vi "Model.vi"(7 "Throttle":dbl, 8 "Turbulance":bool, 9 "dt (s)":dbl=1.0 format="%0.2f", 10 "Motor 4":dbl=-2e-06, 11 "Motor 2":dbl=-2e-06) -> (2 "Position":cluster{"X":dbl, "Y":dbl, "Z":dbl}={"X"=0.0, "Y"=0.0, "Z"=-100.0}, 3 "Angle (degs)":dbl)   [LabVIEW 2011]
uses:
  <vilib>/ptbypt/NI_PtbyPt.lvlib
panel:
  out "M4 Torque":dbl(knob) scale=0.0..3.0
  out "M2 Torque":dbl(knob) scale=0.0..3.0
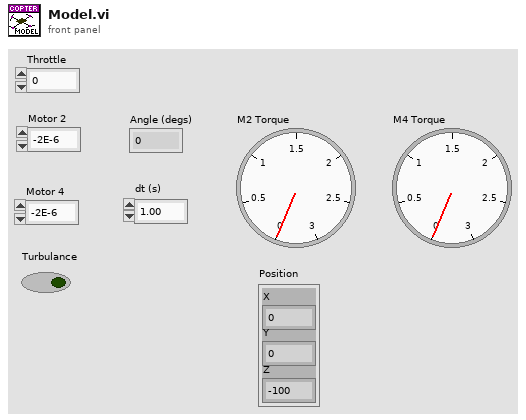
[diagram p1: front panel]
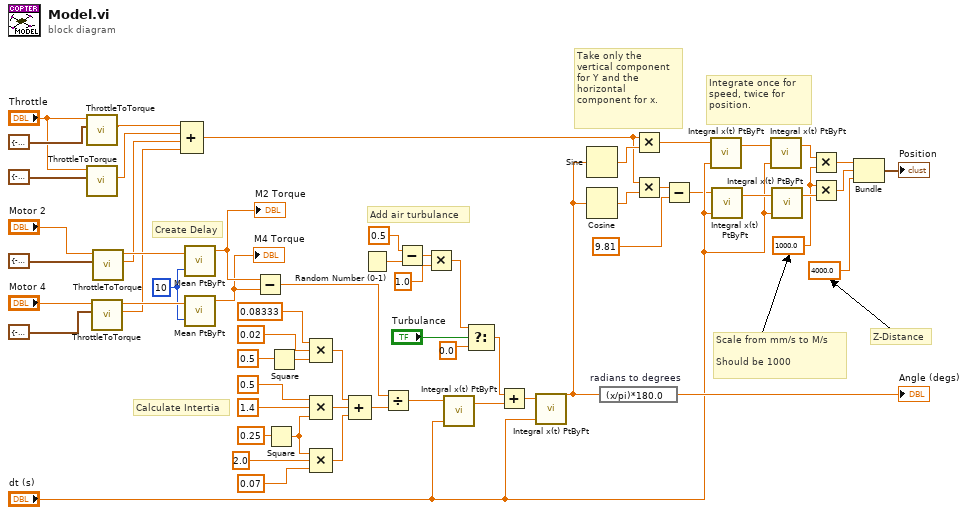
[diagram p0: block diagram]
diagram:
  w10 = 1000.0 ("x*y")
  w36 = 10 ("sample length")
  # "Calculate Intertia"
  # "Add air turbulance"
  # "Integrate once for speed, twice for position."
  # "Take only the vertical component for Y and the horizontal component for x."
  # "Z-Distance"
  # "Scale from mm/s to M/s\n\nShould be 1000"
  # "Create Delay"
  n1 = call "ThrottleToTorque.vi"("Coeffecients"=cluster{"X3":dbl, "X2":dbl, "X1":dbl, "C":dbl} {"X3"=-2.3e-06, "X2"=0.00383, "X1"=-0.639, "C"=49.9}, "Throttle"="Throttle") -> ("Newtons"=w28:dbl)  [unwired: 8 in, 1 out]
  n2 = call "ThrottleToTorque.vi"("Coeffecients"=cluster{"X3":dbl, "X2":dbl, "X1":dbl, "C":dbl} {"X3"=-2.3e-06, "X2"=0.00383, "X1"=-0.639, "C"=49.9}, "Throttle"="Throttle") -> ("Newtons"=w27:dbl)  [unwired: 8 in, 1 out]
  n3 = call "ThrottleToTorque.vi"("Coeffecients"=cluster{"X3":dbl, "X2":dbl, "X1":dbl, "C":dbl} {"X3"=-2.3e-06, "X2"=0.00383, "X1"=-0.639, "C"=49.9} ("Coeffecients 4"), "Throttle"="Motor 4") -> ("Newtons"=w32:dbl, "Torque"=w38:dbl)  [unwired: 8 in]
  n4 = call "ThrottleToTorque.vi"("Coeffecients"=cluster{"X3":dbl, "X2":dbl, "X1":dbl, "C":dbl} {"X3"=-1.671e-06, "X2"=0.003014, "X1"=-0.4197, "C"=12.75} ("Coeffecients 2"), "Throttle"="Motor 2") -> ("Newtons"=w33:dbl, "Torque"=w37:dbl)  [unwired: 8 in]
  n5 = Compound Arithmetic op=ADD(w28, w27, w33, w32) -> (w18:dbl)
  n6 = call <vilib>:"Mean PtByPt.vi"("x"=w37, "sample length"=w36) -> ("mean"=w35:dbl)  [unwired: 2 in, 1 out]
  "M2 Torque" <- w35
  n7 = call <vilib>:"Mean PtByPt.vi"("x"=w38, "sample length"=w36) -> ("mean"=w34:dbl)  [unwired: 2 in, 1 out]
  "M4 Torque" <- w34
  n8 = Subtract(x=w35, y=w34) -> (x-y=w39:dbl)
  n9 = Square(x=0.25) -> (x^2=w48:dbl)
  n10 = Square(x=0.5) -> (x^2=w52:dbl)
  n11 = Compound Arithmetic op=MULTIPLY(0.08333 ("value"), 0.02 ("value"), w52) -> (w55:dbl)
  n12 = Compound Arithmetic op=MULTIPLY(0.5 ("value"), 1.4 ("value"), w48) -> (w51:dbl)
  n13 = Compound Arithmetic op=MULTIPLY(w48, 2.0 ("value"), 0.07 ("value")) -> (w50:dbl)
  n14 = Compound Arithmetic op=unknown(w55, w51, w50) -> (w56:dbl)
  n15 = Random Number (0-1)() -> (number: 0 to 1=w7:dbl)
  n16 = Divide(x=w39, y=w56) -> (x/y=w59:dbl)
  n17 = Subtract(x=0.5, y=w7) -> (x-y=w6:dbl)
  n18 = Multiply(x=w6, y=1.0) -> (x*y=w2:dbl)
  n19 = call <vilib>:"Integral x(t) PtByPt.vi"("dt"="dt (s)", "x"=w59) -> ("integral x(t)"=w40:dbl)  [unwired: 2 in, 1 out]
  n20 = Select(t=w2, s="Turbulance", f=0.0) -> (s? t:f=w4:dbl)
  n21 = Add(x=w4, y=w40) -> (x+y=w41:dbl)
  n22 = call <vilib>:"Integral x(t) PtByPt.vi"("dt"="dt (s)", "x"=w41) -> ("integral x(t)"=w26:dbl)  [unwired: 2 in, 1 out]
  n23 = Sine(x=w26) -> (sin(x)=w25:dbl)
  n24 = Cosine(x=w26) -> (cos(x)=w24:dbl)
  n25 = expression code="(x/pi)*180.0" "radians to degrees"(w26) -> (→"Angle (degs)":dbl)
  n26 = Multiply(x=w18, y=w25) -> (x*y=w23:dbl)
  n27 = Multiply(x=w18, y=w24) -> (x*y=w17:dbl)
  n28 = Subtract(x=w17, y=9.81) -> (x-y=w16:dbl)
  n29 = call <vilib>:"Integral x(t) PtByPt.vi"("dt"="dt (s)", "x"=w23) -> ("integral x(t)"=w21:dbl)  [unwired: 2 in, 1 out]
  n30 = call <vilib>:"Integral x(t) PtByPt.vi"("dt"="dt (s)", "x"=w16) -> ("integral x(t)"=w22:dbl)  [unwired: 2 in, 1 out]
  n31 = call <vilib>:"Integral x(t) PtByPt.vi"("dt"="dt (s)", "x"=w21) -> ("integral x(t)"=w11:dbl)  [unwired: 2 in, 1 out]
  n32 = call <vilib>:"Integral x(t) PtByPt.vi"("dt"="dt (s)", "x"=w22) -> ("integral x(t)"=w13:dbl)  [unwired: 2 in, 1 out]
  n33 = Multiply(x=w11, y=w10) -> (x*y=w14:dbl)
  n34 = Multiply(x=w10, y=w13) -> (x*y=w12:dbl)
  n35 = Bundle(w14, w12, "x*y"=4000.0) -> (→"Position":cluster{dbl, dbl, "x*y":dbl})  [unwired: 1 in]
